vi "error handler.vi"(7 "function (unspecified)":T1, 8 "error in (no error)":errorcluster, 11 "errno":T2) -> (0 "error out":errorcluster)   [LabVIEW 2013, in "Linux RT IPC.C.lvlib"]
uses:
  Linux RT IPC.C.lvlib
  <vilib>/NI/NI Linux RT Errno/Controls/Public/errno.ctl
  Controls/functions.ctl
  <vilib>/NI/NI Linux RT Errno/Linux Errno.lvlib
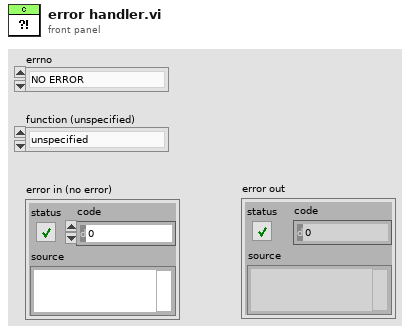
[diagram p1: front panel]
types:
  T1 = typedef "Linux RT IPC.C.lvlib/functions.ctl" = enum16{"unspecified", "close", "fstat", "ftruncate", "mkfifo", "mmap", "munmap", "open", "read", "shm_open", "shm_unlink", "timerfd_create", "timerfd_settime", "timerfd_gettime", "write", "unlink"}
  T2 = typedef "Linux Errno.lvlib/errno.ctl" = enum16{"NO ERROR", "EPERM", "ENOENT", "ESRCH", "EINTR", "EIO", "ENXIO", "E2BIG", "ENOEXEC", "EBADF", "ECHILD", "EAGAIN", "ENOMEM", "EACCES", "EFAULT", "ENOTBLK", "EBUSY", "EEXIST", "EXDEV", "ENODEV", "ENOTDIR", "EISDIR", "EINVAL", "ENFILE", "EMFILE", "ENOTTY", "ETXTBSY", "EFBIG", "ENOSPC", "ESPIPE", "EROFS", "EMLINK", "EPIPE", "EDOM", "ERANGE", "EDADLK", "ENAMETOOLONG", "ENOLCK", "ENOSYS", "ENOTEMPTY", "ELOOP", "EWOULDBLOCK", "ENOMSG", "EIDRM", "ECHRNG", "EL2NSYNC", "EL3HLT", "EL3RST", "ELNRNG", "EUNATCH", "ENOCSI", "EL2HLT", "EBADE", "EBADR", "EXFULL", "ENOANO", "EBADRQC", "EBADSLT", "EDEADLOCK", "EBFONT", "ENOSTR", "ENODATA", "ETIME", "ENOSR", "ENONET", "ENOPKG", "EREMOTE", "ENOLINK", "EADV", "ESRMNT", "ECOMM", "EPROTO", "EMULTIHOP", "EDOTDOT", "EBADMSG", "EOVERFLOW", "ENOTUNIQ", "EBADFD", "EREMCHG", "ELIBACC", "ELIBBAD", "ELIBSCN", "ELIBMAX", "ELIBEXEC", "ELISEQ", "ERESTART", "ESTRPIPE", "EUSERS", "ENOTSOCK", "EDESTADDRREQ", "EMSGSIZE", "EPROTOTYPE", "ENOPROTOOPT", "EPROTONOSUPPORT", "ESOCKTNOSUPPORT", "EOPNOTSUPP", "EPFNOSUPPORT", "EAFNOSUPPORT", "EADDRINUSE", "EADDRNOTAVAIL", "ENETDOWN", "ENETUNREACH", "ENETRESET", "ECONNABORTED", "ECONNRESET", "ENOBUFS", "EISCONN", "ENOTCONN", "ESHUTDOWN", "ETOOMANYREFS", "ETIMEDOUT", "ECONNREFUSED", "EHOSTDOWN", "EHOSTUNREACH", "EALREADY", "EINPROGRESS", "ESTALE", "EUCLEAN", "ENOTNAM", "ENAVAIL", "EISNAM", "EREMOTEIO", "EDQUOT", "ENOMEDIUM", "EMEDIUMTYPE", "ECANCELED", "ENOKEY", "EKEYEXPIRED", "EKEYREVOKED", "EKEYREJECTED", "EOWNERDEAD", "ENOTRECOVERABLE", "ERFKILL", "EHWPOISON", "UNDEFINED"}
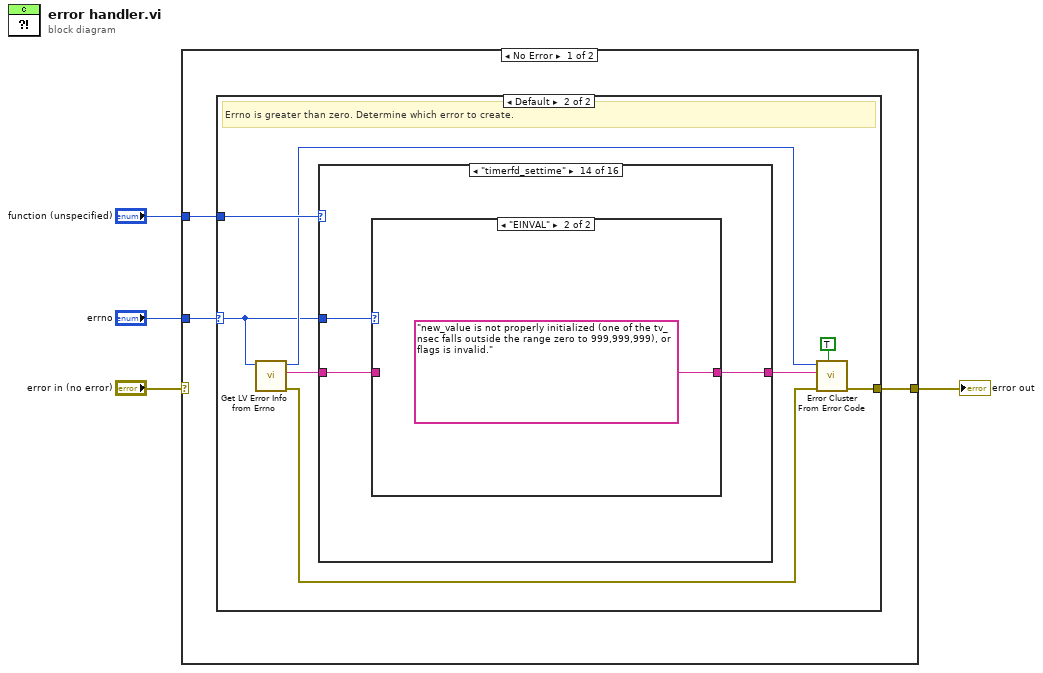
[diagram p0: block diagram]
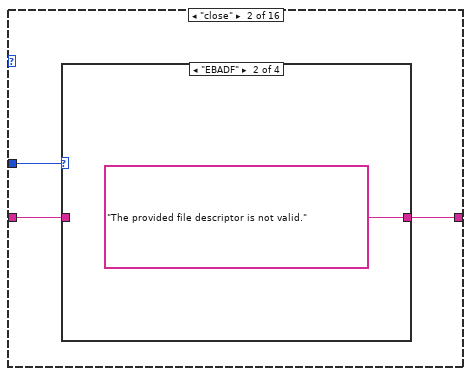
[diagram p4: hidden frame]
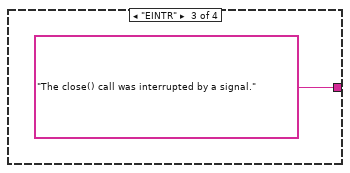
[diagram p6: hidden frame]
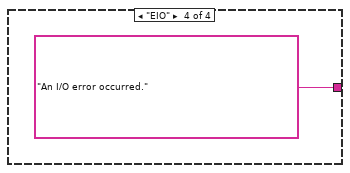
[diagram p7: hidden frame]
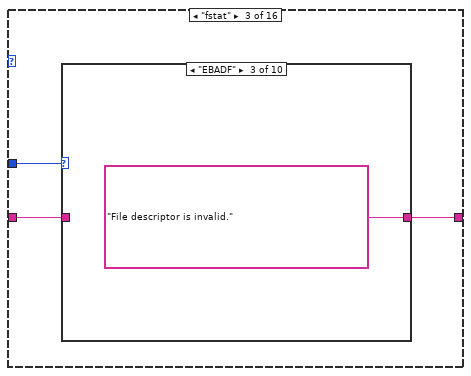
[diagram p8: hidden frame]
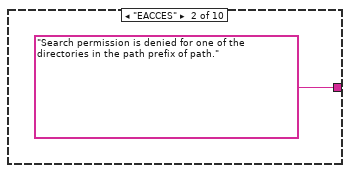
[diagram p10: hidden frame]
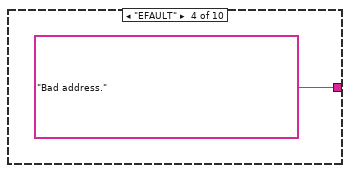
[diagram p11: hidden frame]
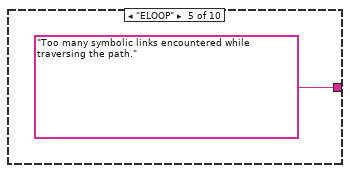
[diagram p12: hidden frame]
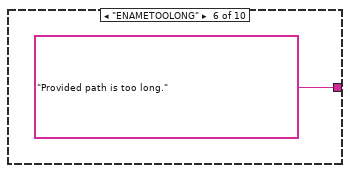
[diagram p13: hidden frame]
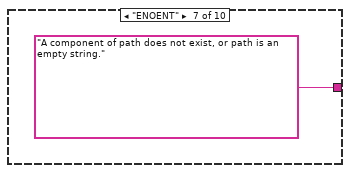
[diagram p14: hidden frame]
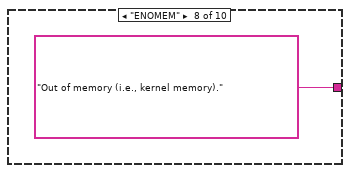
[diagram p15: hidden frame]
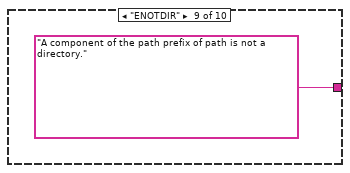
[diagram p16: hidden frame]
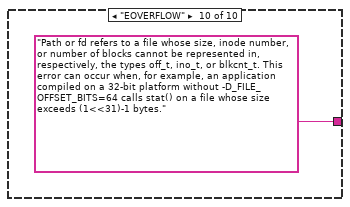
[diagram p17: hidden frame]
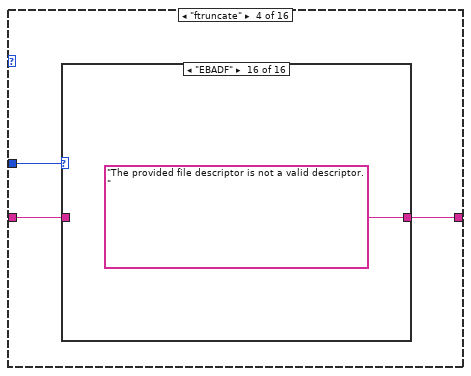
[diagram p18: hidden frame]
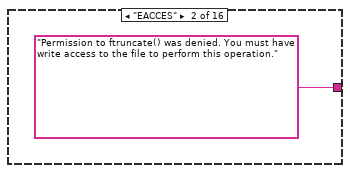
[diagram p20: hidden frame]
diagram:
  n1 = case shown="No Error" "error in (no error)" {
    selector: "error in (no error)" -> [_ w196]
    tunnel: [w7 w196] -> w3
    tunnel: "errno" -> [w5 _]
    tunnel: "function (unspecified)" -> [w6 _]
    frame No Error {
      n2 = case shown="Default" w5 {
        selector: w5 -> [_ w8]
        tunnel: [_ w15] -> w7
        tunnel: w6 -> [_ w13]
        frame "NO ERROR" {
          # "Errno is zero. No error occurred."
        }
        frame Default {
          # "Errno is greater than zero. Determine which error to create."
          n3 = call <vilib>:"Get LV Error Info from Errno.vi"("errno"=w8) -> ("error out"=w9:errorcluster, "error description"=w10:string, "error code"=w11:i32)  [unwired: 8 in]
          n4 = case shown="\"timerfd_settime\"" w13 {
            tunnel: w8 -> [_ w19 w24 w37 w58 w70 w83 w90 w117 w127 w138 w144 w153 w160 w167 w183]
            tunnel: [w16 w18 w26 w39 w57 w68 w84 w89 w116 w129 w140 w146 w155 w162 w166 w182] -> w12
            tunnel: w10 -> [w16 w17 w25 w38 w56 w69 w82 w88 w115 w128 w139 w145 w154 w161 w165 w181]
            frame "unspecified", Default {
              # "No specific function was specified, so use generic error description."
            }
            frame "close" {
              n5 = case shown="\"EBADF\"" w19 {
                tunnel: [w20 "The provided file descriptor is not valid." "The close() call was interrupted by a signal." "An I/O error occurred."] -> w18
                tunnel: w17 -> [w20 _ _ _]
                frame "NO ERROR", Default {
                }
                frame "EBADF" {
                }
                frame "EINTR" {
                }
                frame "EIO" {
                }
              }
            }
            frame "fstat" {
              n6 = case shown="\"EBADF\"" w24 {
                tunnel: [w27 "Search permission is denied for one of the directories in the path prefix of path." "File descriptor is invalid." "Bad address." "Too many symbolic links encountered while traversing the path." "Provided path is too long." "A component of path does not exist, or path is an empty string." "Out of memory (i.e., kernel memory)." "A component of the path prefix of path is not a directory." "Path or fd refers to a file whose size, inode number, or number of blocks cannot be represented in, respectively, the types off_t, ino_t, or blkcnt_t. This error can occur when, for example, an application compiled on a 32-bit platform without -D_FILE_OFFSET_BITS=64 calls stat() on a file whose size exceeds (1<<31)-1 bytes."] -> w26
                tunnel: w25 -> [w27 _ _ _ _ _ _ _ _ _]
                frame "NO ERROR", Default {
                }
                frame "EACCES" {
                }
                frame "EBADF" {
                }
                frame "EFAULT" {
                }
                frame "ELOOP" {
                }
                frame "ENAMETOOLONG" {
                }
                frame "ENOENT" {
                }
                frame "ENOMEM" {
                }
                frame "ENOTDIR" {
                }
                frame "EOVERFLOW" {
                }
              }
            }
            frame "ftruncate" {
              n7 = case shown="\"EBADF\"" w37 {
                tunnel: [w40 "Permission to ftruncate() was denied. You must have write access to the file to perform this operation." "The requested size is larger than the maximum file size." "While blocked waiting to complete, the call was interrupted by a signal handler." "The file descriptor does not reference a regular file." "An I/O error occurred updating the inode." "The named file is a directory." "Too many symbolic links were encountered in translating the pathname." "The length of name exceeds PATH_MAX." "The system-wide limit on the total number of open files has been reached." "The named file does not exist." "A component of the path prefix is not a directory." "The underlying file system does not support extending a file beyond its current size." "The named file resides on a read-only file system." "The file is a pure procedure (shared text) file that is being executed." "The provided file descriptor is not a valid descriptor."] -> w39
                tunnel: w38 -> [w40 _ _ _ _ _ _ _ _ _ _ _ _ _ _ _]
                frame "NO ERROR", Default {
                }
                frame "EACCES" {
                }
                frame "EFBIG" {
                }
                frame "EINTR" {
                }
                frame "EINVAL" {
                }
                frame "EIO" {
                }
                frame "EISDIR" {
                }
                frame "ELOOP" {
                }
                frame "ENAMETOOLONG" {
                }
                frame "ENFILE" {
                }
                frame "ENOENT" {
                }
                frame "ENOTDIR" {
                }
                frame "EPERM" {
                }
                frame "EROFS" {
                }
                frame "ETXTBSY" {
                }
                frame "EBADF" {
                }
              }
            }
            frame "mkfifo" {
              n8 = case shown="\"EACCES\"" w58 {
                tunnel: [w59 "One of the directories in pathname did not allow search (execute) permission." "The user's quota of disk blocks or inodes on the file system has been exhausted." "pathname already exists. This includes the case where pathname is a symbolic link, dangling or not." "Either the total length of pathname is greater than PATH_MAX, or an individual filename component has a length greater than NAME_MAX. In the GNU system, there is no imposed limit on overall filename length, but some file systems may place limits on the length of a component." "A directory component in pathname does not exist or is a dangling symbolic link." "The directory or file system has no room for the new file." "A component used as a directory in pathname is not, in fact, a directory." "pathname refers to a read-only file system."] -> w57
                tunnel: w56 -> [w59 _ _ _ _ _ _ _ _]
                frame "NO ERROR", Default {
                }
                frame "EACCES" {
                }
                frame "EDQUOT" {
                }
                frame "EEXIST" {
                }
                frame "ENAMETOOLONG" {
                }
                frame "ENOENT" {
                }
                frame "ENOSPC" {
                }
                frame "ENOTDIR" {
                }
                frame "EROFS" {
                }
              }
            }
            frame "mmap" {
              n9 = case shown="\"EACCES\"" w70 {
                tunnel: [w71 "File access/permission error. The cause of the error is due to one of the following reasons:\n1. A file descriptor refers to a non-regular file.\n2. A file mapping was requested, but the file descriptor is not open for reading.\n3. Mapping for a shared process was requested and and write access is requested, but the file descriptor is not open in read/write mode.\n4. Write access is requested, but the file is append-only." "The file has been locked, or too much memory has been locked." "The file descriptor is not a valid file descriptor (and MAP_ANONYMOUS was not set)." "An input parameter to mmap() was invalid. Possible issues are:\n1. The requested length was zero (nothing to map).\n2. The offset was not a multiple of the system's page size (and therefore wasn't lined up on a page boundary).\n3. flags contained neither MAP_PRIVATE or MAP_SHARED, or contained both of these values." "The system-wide limit on the total number of open files has been reached." "The underlying filesystem of the specified file does not support memory mapping." "No memory is available. The process's maximum number of mappings could have been exceeded." "The prot argument asks for PROT_EXEC but the mapped area belongs to a file on a filesystem that was mounted no-exec. Or, the operation was prevented by a file seal." "MAP_DENYWRITE was set but the object specified by fd is open for writing." "On 32-bit architecture together with the large file extension (i.e., using 64-bit off_t): the number of pages used for length plus number of pages used for offset would overflow unsigned long (32 bits)."] -> w68
                tunnel: w69 -> [w71 _ _ _ _ _ _ _ _ _ _]
                frame "NO ERROR", Default {
                }
                frame "EACCES" {
                }
                frame "EAGAIN" {
                }
                frame "EBADF" {
                }
                frame "EINVAL" {
                }
                frame "ENFILE" {
                }
                frame "ENODEV" {
                }
                frame "ENOMEM" {
                }
                frame "EPERM" {
                }
                frame "ETXTBSY" {
                }
                frame "EOVERFLOW" {
                }
              }
            }
            frame "munmap" {
              n10 = case shown="\"EINVAL\"" w83 {
                tunnel: [w85 "An input parameter to munmap() was invalid. Possible issues are:\nLength of memory to unmap was zero." "No memory is available. This error can occur for munmap() if unmapping is attempted while the same region in memory is being mapped concurrently."] -> w84
                tunnel: w82 -> [w85 _ _]
                frame "NO ERROR", Default {
                }
                frame "EINVAL" {
                }
                frame "ENOMEM" {
                }
              }
            }
            frame "open" {
              n11 = case shown="\"EWOULDBLOCK\"" w90 {
                tunnel: [w91 "The requested access to the file is not allowed, or search permission is denied for one of the directories in the path prefix of pathname, or the file did not exist yet and write access to the parent directory is not allowed." "Where O_CREAT is specified, the file does not exist, and the user's quota of disk blocks or inodes on the file system has been exhausted." "pathname already exists and O_CREAT and O_EXCL were used." "pathname points outside your accessible address space." "pathname refers to a regular file that is too large to be opened. The usual scenario here is that an application compiled on a 32-bit platform without -D_FILE_OFFSET_BITS=64 tried to open a file whose size exceeds (2<<31)-1 bits." "While blocked waiting to complete, the call was interrupted by a signal handler." "The file descriptor does not reference a regular file." "pathname refers to a directory and the access requested involved writing (that is, O_WRONLY or O_RDWR is set)." "Too many symbolic links were encountered in resolving pathname." "The process already has the maximum number of files open." "pathname was too long." "The system limit on the total number of open files has been reached." "pathname refers to a device special file and no corresponding device exists." "The named file does not exist." "Insufficient kernel memory was available." "pathname was to be created but the device containing pathname has no room for the new file." "A component used as a directory in pathname is not, in fact, a directory." "O_NONBLOCK | O_WRONLY is set, the named file is a FIFO and no process has the file open for reading. Or, the file is a device special file and no corresponding device exists." "pathname refers to a regular file that is too large to be opened. The usual scenario here is that an application compiled on a 32-bit platform without -D_FILE_OFFSET_BITS=64 tried to open a file whose size exceeds (2<<31)-1 bits." "The O_NOATIME flag was specified, but the effective user ID of the caller did not match the owner of the file and the caller was not privileged (CAP_FOWNER)." "pathname refers to a file on a read-only file system and write access was requested." "pathname refers to an executable image which is currently being executed and write access was requested." "The O_NONBLOCK flag was specified, and an incompatible lease was held on the file."] -> w89
                tunnel: w88 -> [w91 _ _ _ _ _ _ _ _ _ _ _ _ _ _ _ _ _ _ _ _ _ _ _]
                frame "NO ERROR", Default {
                }
                frame "EACCES" {
                }
                frame "EDQUOT" {
                }
                frame "EEXIST" {
                }
                frame "EFAULT" {
                }
                frame "EFBIG" {
                }
                frame "EINTR" {
                }
                frame "EINVAL" {
                }
                frame "EISDIR" {
                }
                frame "ELOOP" {
                }
                frame "EMFILE" {
                }
                frame "ENAMETOOLONG" {
                }
                frame "ENFILE" {
                }
                frame "ENODEV" {
                }
                frame "ENOENT" {
                }
                frame "ENOMEM" {
                }
                frame "ENOSPC" {
                }
                frame "ENOTDIR" {
                }
                frame "ENXIO" {
                }
                frame "EOVERFLOW" {
                }
                frame "EPERM" {
                }
                frame "EROFS" {
                }
                frame "ETXTBSY" {
                }
                frame "EWOULDBLOCK" {
                }
              }
            }
            frame "read" {
              n12 = case shown="\"EINVAL\"" w117 {
                tunnel: [w118 "The file descriptor fd refers to a file other than a socket and has been marked nonblocking (O_NONBLOCK), and the read would block." "The file descriptor fd refers to a file other than a socket and has been marked nonblocking (O_NONBLOCK), and the read would block." "fd is not a valid file descriptor or is not open for reading." "buf is outside your accessible address space." "The call was interrupted by a signal before any data was read" "fd is attached to an object which is unsuitable for reading; or the file was opened with the O_DIRECT flag, and either the address specified in buf, the value specified in count, or the current file offset is not suitably aligned." "An I/O error occurred." "fd refers to a directory."] -> w116
                tunnel: w115 -> [w118 _ _ _ _ _ _ _ _]
                frame "NO ERROR", Default {
                }
                frame "EAGAIN" {
                }
                frame "EWOULDBLOCK" {
                }
                frame "EBADF" {
                }
                frame "EFAULT" {
                }
                frame "EINTR" {
                }
                frame "EINVAL" {
                }
                frame "EIO" {
                }
                frame "EISDIR" {
                }
              }
            }
            frame "shm_open" {
              n13 = case shown="\"ENOENT\"" w127 {
                tunnel: [w130 "Permission was denied to shm_open(). This error can occur when trying to open an existing shared memory file that does not allow read access, or when trying to create or replace a file that does not allow write access." "shm_open() tried to create a shared memory file, but the file already existed." "The name argument to shm_open() was invalid." "The per-process limit on the number of open file descriptors has been reached. This can occur if file references are being opened and not being closed." "The length of name exceeds PATH_MAX. Shorten the shared memory name." "The system-wide limit on the total number of open files has been reached." "An attempt was made to shm_open() a shared memory name that did not exist, and the create flag was not specified."] -> w129
                tunnel: w128 -> [w130 _ _ _ _ _ _ _]
                frame "NO ERROR", Default {
                }
                frame "EACCES" {
                }
                frame "EEXIST" {
                }
                frame "EINVAL" {
                }
                frame "EMFILE" {
                }
                frame "ENAMETOOLONG" {
                }
                frame "ENFILE" {
                }
                frame "ENOENT" {
                }
              }
            }
            frame "shm_unlink" {
              n14 = case shown="\"EACCES\"" w138 {
                tunnel: [w141 "Permission to shm_unlink() the shared memory object was denied." "An attempt was to made to shm_unlink() a filename that does not exist."] -> w140
                tunnel: w139 -> [w141 _ _]
                frame "NO ERROR", Default {
                }
                frame "EACCES" {
                }
                frame "ENOENT" {
                }
              }
            }
            frame "timerfd_create" {
              n15 = case shown="\"ENOMEM\"" w144 {
                tunnel: [w147 "The clockid argument is neither CLOCK_MONOTONIC nor CLOCK_REALTIME, or flags is invalid." "The per-process limit on the number of open file descriptors has been reached." "The system-wide limit on the total number of open files has been reached." "Could not mount (internal) anonymous inode device." "There was insufficient kernel memory to create the timer."] -> w146
                tunnel: w145 -> [w147 _ _ _ _ _]
                frame "NO ERROR", Default {
                }
                frame "EINVAL" {
                }
                frame "EMFILE" {
                }
                frame "ENFILE" {
                }
                frame "ENODEV" {
                }
                frame "ENOMEM" {
                }
              }
            }
            frame "timerfd_gettime" {
              n16 = case shown="\"EFAULT\"" w153 {
                tunnel: [w156 "fd is not a valid timerfd file descriptor." "fd is not a valid file descriptor." "new_value, old_value, or curr_value is not valid a pointer."] -> w155
                tunnel: w154 -> [w156 _ _ _]
                frame "NO ERROR", Default {
                }
                frame "EINVAL" {
                }
                frame "EBADF" {
                }
                frame "EFAULT" {
                }
              }
            }
            frame "timerfd_settime" {
              n17 = case shown="\"EINVAL\"" w160 {
                tunnel: [w163 "new_value is not properly initialized (one of the tv_nsec falls outside the range zero to 999,999,999), or flags is invalid."] -> w162
                tunnel: w161 -> [w163 _]
                frame "NO ERROR", Default {
                }
                frame "EINVAL" {
                }
              }
            }
            frame "unlink" {
              n18 = case shown="\"EIO\"" w167 {
                tunnel: [w168 "Write access to the directory containing pathname is not allowed for the process's effective UID, or one of the directories in pathname did not allow search permission." "The file pathname cannot be unlinked because it is being used by the system or another process." "pathname points outside your accessible address space." "An I/O error occurred." "pathname refers to a directory." "Too many symbolic links were encountered in translating pathname." "pathname was too long." "A component in pathname does not exist or is a dangling symbolic link, or pathname is empty." "Insufficient kernel memory was available." "A component used as a directory in pathname is not, in fact, a directory." "The system does not allow unlinking of directories, or unlinking of directories requires privileges that the calling process doesn't have. Or, the file system does not allow unlinking of files." "pathname refers to a file on a read-only file system."] -> w166
                tunnel: w165 -> [w168 _ _ _ _ _ _ _ _ _ _ _ _]
                frame "NO ERROR", Default {
                }
                frame "EACCES" {
                }
                frame "EBUSY" {
                }
                frame "EFAULT" {
                }
                frame "EIO" {
                }
                frame "EISDIR" {
                }
                frame "ELOOP" {
                }
                frame "ENAMETOOLONG" {
                }
                frame "ENOENT" {
                }
                frame "ENOMEM" {
                }
                frame "ENOTDIR" {
                }
                frame "EPERM" {
                }
                frame "EROFS" {
                }
              }
            }
            frame "write" {
              n19 = case shown="\"EPIPE\"" w183 {
                tunnel: [w184 "The file descriptor fd refers to a file other than a socket and has been marked nonblocking (O_NONBLOCK), and the write would block." "The file descriptor fd refers to a file other than a socket and has been marked nonblocking (O_NONBLOCK), and the write would block." "fd is not a valid file descriptor or is not open for writing." "fd refers to a datagram socket for which a peer address has not been set using connect(2)." "The user's quota of disk blocks on the file system containing the file referred to by fd has been exhausted." "buf is outside your accessible address space." "An attempt was made to write a file that exceeds the implementation-defined maximum file size or the process's file size limit, or to write at a position past the maximum allowed offset." "The call was interrupted by a signal before any data was written." "A low-level I/O error occurred while modifying the inode." "The device containing the file referred to by fd has no room for the data." "fd is connected to a pipe or socket whose reading end is closed. When this happens the writing process will also receive a SIGPIPE signal. (Thus, the write return value is seen only if the program catches, blocks or ignores this signal.)"] -> w182
                tunnel: w181 -> [w184 _ _ _ _ _ _ _ _ _ _ _]
                frame "NO ERROR", Default {
                }
                frame "EAGAIN" {
                }
                frame "EWOULDBLOCK" {
                }
                frame "EBADF" {
                }
                frame "EDESTADDRREQ" {
                }
                frame "EDQUOT" {
                }
                frame "EFAULT" {
                }
                frame "EFBIG" {
                }
                frame "EINTR" {
                }
                frame "EIO" {
                }
                frame "ENOSPC" {
                }
                frame "EPIPE" {
                }
              }
            }
          }
          n20 = call <vilib>:"Error Cluster From Error Code.vi"("show call chain? (False)"=TRUE, "error in (no error)"=w9, "error message (\"\")"=w12, "error code (0)"=w11) -> ("error out"=w15:errorcluster)  [unwired: 5 in]
        }
      }
    }
    frame Error {
      # "Error already exists. Pass through."
    }
  }
  "error out" <- w3
